vi "RSZVB Set Calibration Reference Plane Shift Specific.vi"(7 "Calibration Name (\"\")":string, 8 "error in (no error)":errorcluster {"code" format="%.0x"}, 9 "Reference Plane Shift (0.0)":dbl format="%^.3e", 10 "Channel (1)":i32=1, 11 "VISA resource name":refnum<visa-resource-name>) -> (0 "error out":errorcluster {"code" format="%.0x"}, 3 "VISA resource name out":refnum<visa-resource-name>)   [LabVIEW 2011]
doc: "This VI specifies the reference plane shift that is applied to the specified calibration only.\n\nRemote-control command(s):\n[SENSe<Ch>:]CORRection:COLLect:RPSHift"
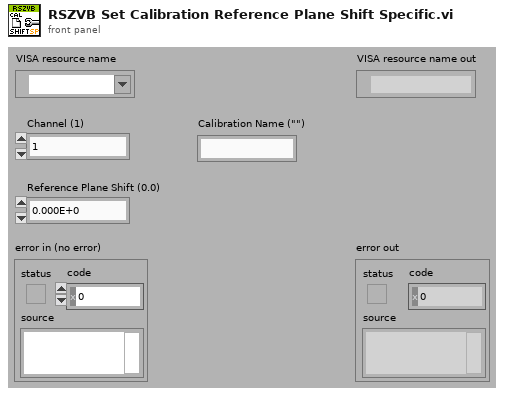
[diagram p1: front panel]
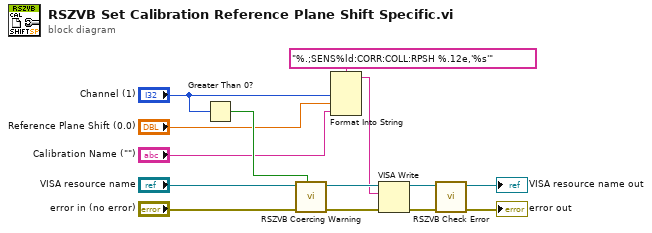
[diagram p0: block diagram]
diagram:
  n1 = Greater Than 0?(x="Channel (1)") -> (x > 0?=w8:bool)
  n2 = call "RSZVB Coercing Warning.vi"("In Range?"=w8, "error in (no error)"="error in (no error)", "VISA session"="VISA resource name") -> ("error out"=w12:errorcluster, "dup VISA session"=w13:refnum<visa-resource-name>)  [unwired: 7 in]
  n3 = Format Into String(format string="%.;SENS%ld:CORR:COLL:RPSH %.12e,'%s'", "Channel (1)", "Reference Plane Shift (0.0)", "Calibration Name (\"\")") -> (resulting string=w9:string)  [unwired: 2 in, 1 out]
  n4 = VISA Write(VISA resource name=w13, write buffer=w9, error in (no error)=w12) -> (VISA resource name out=w10:refnum<visa-resource-name>, error out=w11:errorcluster)  [unwired: 1 out]
  n5 = call "RSZVB Check Error.vi"("error in (no error)"=w11, "VISA session"=w10) -> ("error out"=→"error out":errorcluster, "dup VISA session"=→"VISA resource name out":refnum<visa-resource-name>)  [unwired: 8 in]
